vi "Initialize Hardware.vi"(8 "error in (no error)":errorcluster, 9 "DAQ Type":enum16{"Hardware", "Simulation"}(ring), 10 "Connection Ref":variant, 11 "Agilent 3054A in":refnum<class "Agilent 3054A.lvclass">) -> (0 "error out":errorcluster, 3 "Agilent 3054A out":refnum<class "Agilent 3054A.lvclass">)   [LabVIEW 2016, in "Oscilloscope.lvlib" / "Agilent 3054A.lvclass"]
uses:
  Agilent 3054A.lvclass
  Agilent 3054A.lvclass/Agilent 3054A.ctl
  <instrlib>/Agilent 2000 3000 X-Series/Agilent 2000 3000 X-Series.lvlib
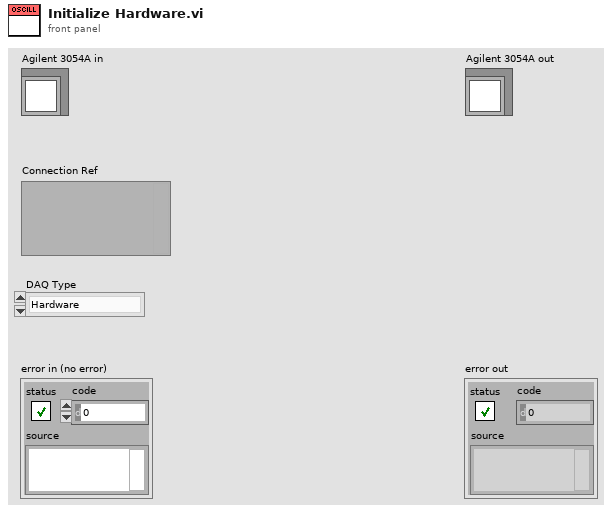
[diagram p1: front panel]
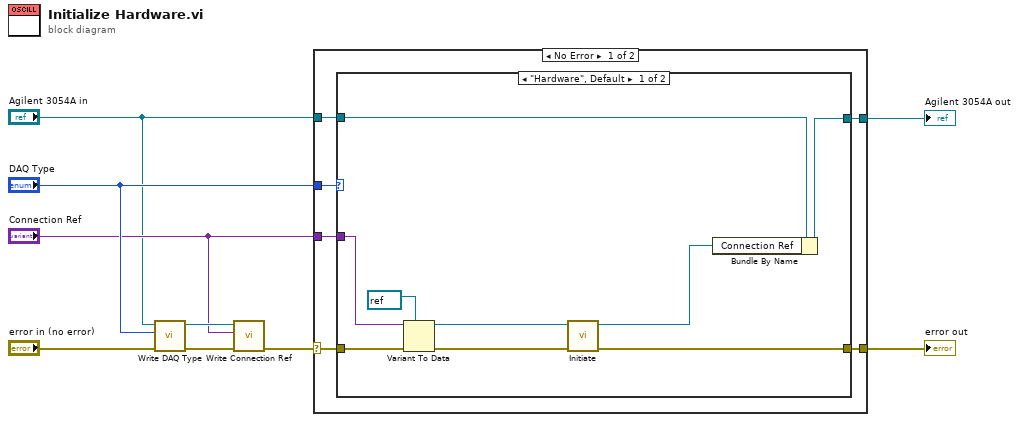
[diagram p0: block diagram]
diagram:
  n1 = call-dynamic "Write DAQ Type.vi"("error in (no error)"="error in (no error)", "DAQ Type"="DAQ Type", "Agilent 3054A in"="Agilent 3054A in") -> ("error out"=w8:errorcluster, "Agilent 3054A out"=w6:refnum<class "Agilent 3054A.lvclass">)  [unwired: 7 in]
  n2 = call-dynamic "Write Connection Ref.vi"("error in (no error)"=w8, "Connection Ref"="Connection Ref", "Agilent 3054A in"=w6) -> ("error out"=w7:errorcluster)  [unwired: 7 in, 1 out]
  n3 = case shown="No Error" w7 {
    selector: w7 -> [w12 w27]
    tunnel: "DAQ Type" -> [w15 _]
    tunnel: "Connection Ref" -> [w14 _]
    tunnel: "Agilent 3054A in" -> [w13 w28]
    tunnel: [w11 w28] -> w2
    tunnel: [w10 w27] -> w1
    frame No Error {
      n4 = case shown="\"Hardware\", Default" w15 {
        tunnel: w14 -> [w23 _]
        tunnel: w13 -> [w21 w26]
        tunnel: w12 -> [w24 w25]
        tunnel: [w20 w26] -> w11
        tunnel: [w17 w25] -> w10
        frame "Hardware", Default {
          n5 = Variant To Data(error in=w24, type=refnum<visa-resource-name> refnum ("VISA resource name"), Variant=w23) -> (data=w19:refnum<visa-resource-name>, error out=w18:errorcluster)
          n6 = call <instrlib>:"Initiate.vi"("error in (no error)"=w18, "VISA resource name"=w19) -> ("error out"=w17:errorcluster, "VISA resource name out"=w16:refnum<visa-resource-name>)  [unwired: 8 in]
          n7 = Bundle By Name(cluster=w21, "Connection Ref"=w16) -> (w20:refnum<class "Agilent 3054A.lvclass">)
        }
        frame "Simulation" {
        }
      }
    }
    frame Error {
    }
  }
  "error out" <- w1
  "Agilent 3054A out" <- w2
